vi "006 Crear dos arrays 100 posicions.vi"() -> ()   [LabVIEW 2019]
panel:
  out "Random temp":dbl[][](graph)
  in  "TempMax":i32
  in  "TempMin":i32
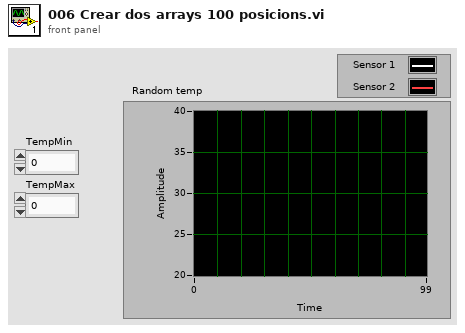
[diagram p1: front panel]
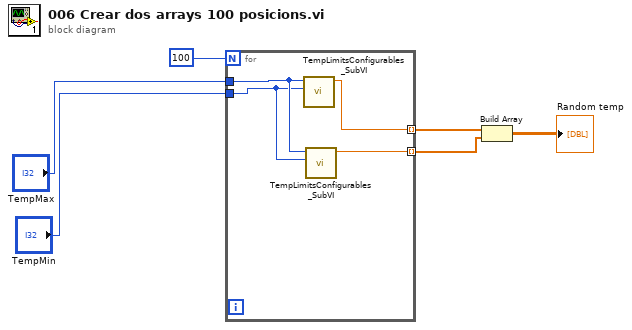
[diagram p0: block diagram]
diagram:
  n1 = for {
    N: 100 -> [_]
    tunnel: "TempMax" -> [w10]
    tunnel: "TempMin" -> [w9]
    tunnel: [w8] -> w3 mode=indexing
    tunnel: [w7] -> w2 mode=indexing
    n2 = call "TempLimitsConfigurables_SubVI.vi"("TempMin"=w9, "TempMax"=w10) -> ("RandomTemp"=w7:dbl)  [unwired: 9 in]
    n3 = call "TempLimitsConfigurables_SubVI.vi"("TempMin"=w9, "TempMax"=w10) -> ("RandomTemp"=w8:dbl)  [unwired: 9 in]
  }
  n4 = Build Array(w2, w3) -> (→"Random temp":dbl[][])
